vi "QBridge 0MQ weather.vi"() -> (0 "error":errorcluster)   [LabVIEW 2018]
uses:
  <vilib>/addons/zeromq/zmq_socket.lvclass
  <vilib>/addons/zeromq/zmq_context.lvclass
  <vilib>/addons/zeromq/socket_type.ctl
  <vilib>/addons/zeromq/socket_options.ctl
  Global_Telescopio.vi
  <vilib>/addons/zeromq/zeromq.lvlib
panel:
  in  "stop":bool
  # "QBRIDGE ZeroMQ \nSUB Weather"
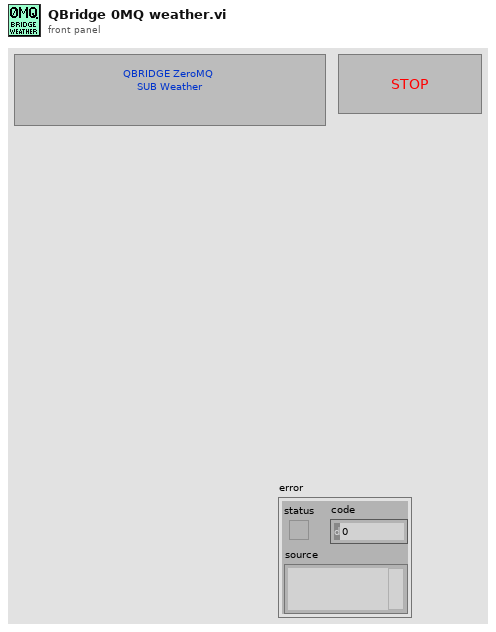
[diagram p1: front panel]
types:
  T1 = typedef "zeromq.lvlib/socket_options.ctl" = enum8{"NONE", "ZMQ_HWM", "<2>", "ZMQ_SWAP", "ZMQ_AFFINITY", "ZMQ_ROUTING_ID", "ZMQ_SUBSCRIBE", "ZMQ_UNSUBSCRIBE", "ZMQ_RATE", "ZMQ_RECOVERY_IVL", "ZMQ_MCAST_LOOP", "ZMQ_SNDBUF", "ZMQ_RCVBUF", "ZMQ_RCVMORE", "ZMQ_FD", "ZMQ_EVENTS", "ZMQ_TYPE", "ZMQ_LINGER", "ZMQ_RECONNECT_IVL", "ZMQ_BACKLOG", "ZMQ_RECOVERY_IVL_MSEC", "ZMQ_RECONNECT_IVL_MAX", "ZMQ_MAXMSGSIZE", "ZMQ_SNDHWM", "ZMQ_RCVHWM", "ZMQ_MULTICAST_HOPS", "<26>", "ZMQ_RCVTIMEO", "ZMQ_SNDTIMEO", "<29>", "<30>", "ZMQ_IPV4ONLY", "ZMQ_LAST_ENDPOINT", "ZMQ_ROUTER_MANDATORY", "ZMQ_TCP_KEEPALIVE", "ZMQ_TCP_KEEPALIVE_CNT", "ZMQ_TCP_KEEPALIVE_IDLE", "ZMQ_TCP_KEEPALIVE_INTVL", "ZMQ_TCP_ACCEPT_FILTER", "ZMQ_IMMEDIATE", "ZMQ_XPUB_VERBOSE", "ZMQ_ROUTER_RAW", "ZMQ_IPV6", "ZMQ_MECHANISM", "ZMQ_PLAIN_SERVER", "ZMQ_PLAIN_USERNAME", "ZMQ_PLAIN_PASSWORD", "ZMQ_CURVE_SERVER", "ZMQ_CURVE_PUBLICKEY", "ZMQ_CURVE_SECRETKEY", "ZMQ_CURVE_SERVERKEY", "ZMQ_PROBE_ROUTER", "ZMQ_REQ_CORRELATE", "ZMQ_REQ_RELAXED", "ZMQ_CONFLATE", "ZMQ_ZAP_DOMAIN", "ZMQ_ROUTER_HANDOVER", "ZMQ_TOS", "ZMQ_IPC_FILTER_PID", "ZMQ_IPC_FILTER_UID", "ZMQ_IPC_FILTER_GID", "ZMQ_CONNECT_ROUTING_ID", "ZMQ_GSSAPI_SERVER", "ZMQ_GSSAPI_PRINCIPAL", "ZMQ_GSSAPI_SERVICE_PRINCIPAL", "ZMQ_GSSAPI_PLAINTEXT", "ZMQ_HANDSHAKE_IVL", "<67>", "ZMQ_SOCKS_PROXY", "ZMQ_XPUB_NODROP", "ZMQ_BLOCKY", "ZMQ_XPUB_MANUAL", "ZMQ_XPUB_WELCOME_MSG", "ZMQ_STREAM_NOTIFY", "ZMQ_INVERT_MATCHING", "ZMQ_HEARTBEAT_IVL", "ZMQ_HEARTBEAT_TTL", "ZMQ_HEARTBEAT_TIMEOUT", "ZMQ_XPUB_VERBOSER", "ZMQ_CONNECT_TIMEOUT", "ZMQ_TCP_MAXRT", "ZMQ_THREAD_SAFE", "<82>", "<83>", "ZMQ_MULTICAST_MAXTPDU", "ZMQ_VMCI_BUFFER_SIZE", "ZMQ_VMCI_BUFFER_MIN_SIZE", "ZMQ_VMCI_BUFFER_MAX_SIZE", "ZMQ_VMCI_CONNECT_TIMEOUT", "ZMQ_USE_FD", "ZMQ_GSSAPI_PRINCIPAL_NAMETYPE", "ZMQ_GSSAPI_SERVICE_PRINCIPAL_NAMETYPE", "ZMQ_BINDTODEVICE", "ZMQ_ZAP_ENFORCE_DOMAIN", "ZMQ_LOOPBACK_FASTPATH", "ZMQ_METADATA", "ZMQ_MULTICAST_LOOP", "ZMQ_ROUTER_NOTIFY"}
  T2 = typedef "zeromq.lvlib/socket_type.ctl" = enum8{"ZMQ_PAIR", "ZMQ_PUB", "ZMQ_SUB", "ZMQ_REQ", "ZMQ_REP", "ZMQ_DEALER", "ZMQ_ROUTER", "ZMQ_PULL", "ZMQ_PUSH", "ZMQ_XPUB", "ZMQ_XSUB", "ZMQ_STREAM", "ZMQ_SERVER", "ZMQ_CLIENT", "ZMQ_RADIO", "ZMQ_DISH", "ZMQ_GATHER", "ZMQ_SCATTER", "ZMQ_DGRAM"}
  T3 = cluster{"broker":string, "version":string, "date":string, "hour":string, "outTemp":string, "hiTemp":string, "lowTemp":string, "outHumidity":string, "dewOut":string, "windSpeed":string, "windDirection":string, "windRun":string, "hiSpeed":string, "hiDir":string, "windChill":string, "heatIndex":string, "THWIndex":string, "THSIndex":string, "pressure":string, "rain":string, "rainRate":string, "solarRad":string, "solarEnergy":string, "hiSolarRad":string, "UVIndex":string, "UVDose":string, "hiUV":string, "headDD":string, "coolDD":string, "inTemp":string, "inHumidity":string, "inHeat":string, "inEMC":string, "inAirDensity":string, "2ndTemp":string, "2ndHumidity":string, "ET":string, "leaf":string, "windSamp":string, "windTx":string, "ISSRecept":string, "dewIn":string, "arcInt":string}
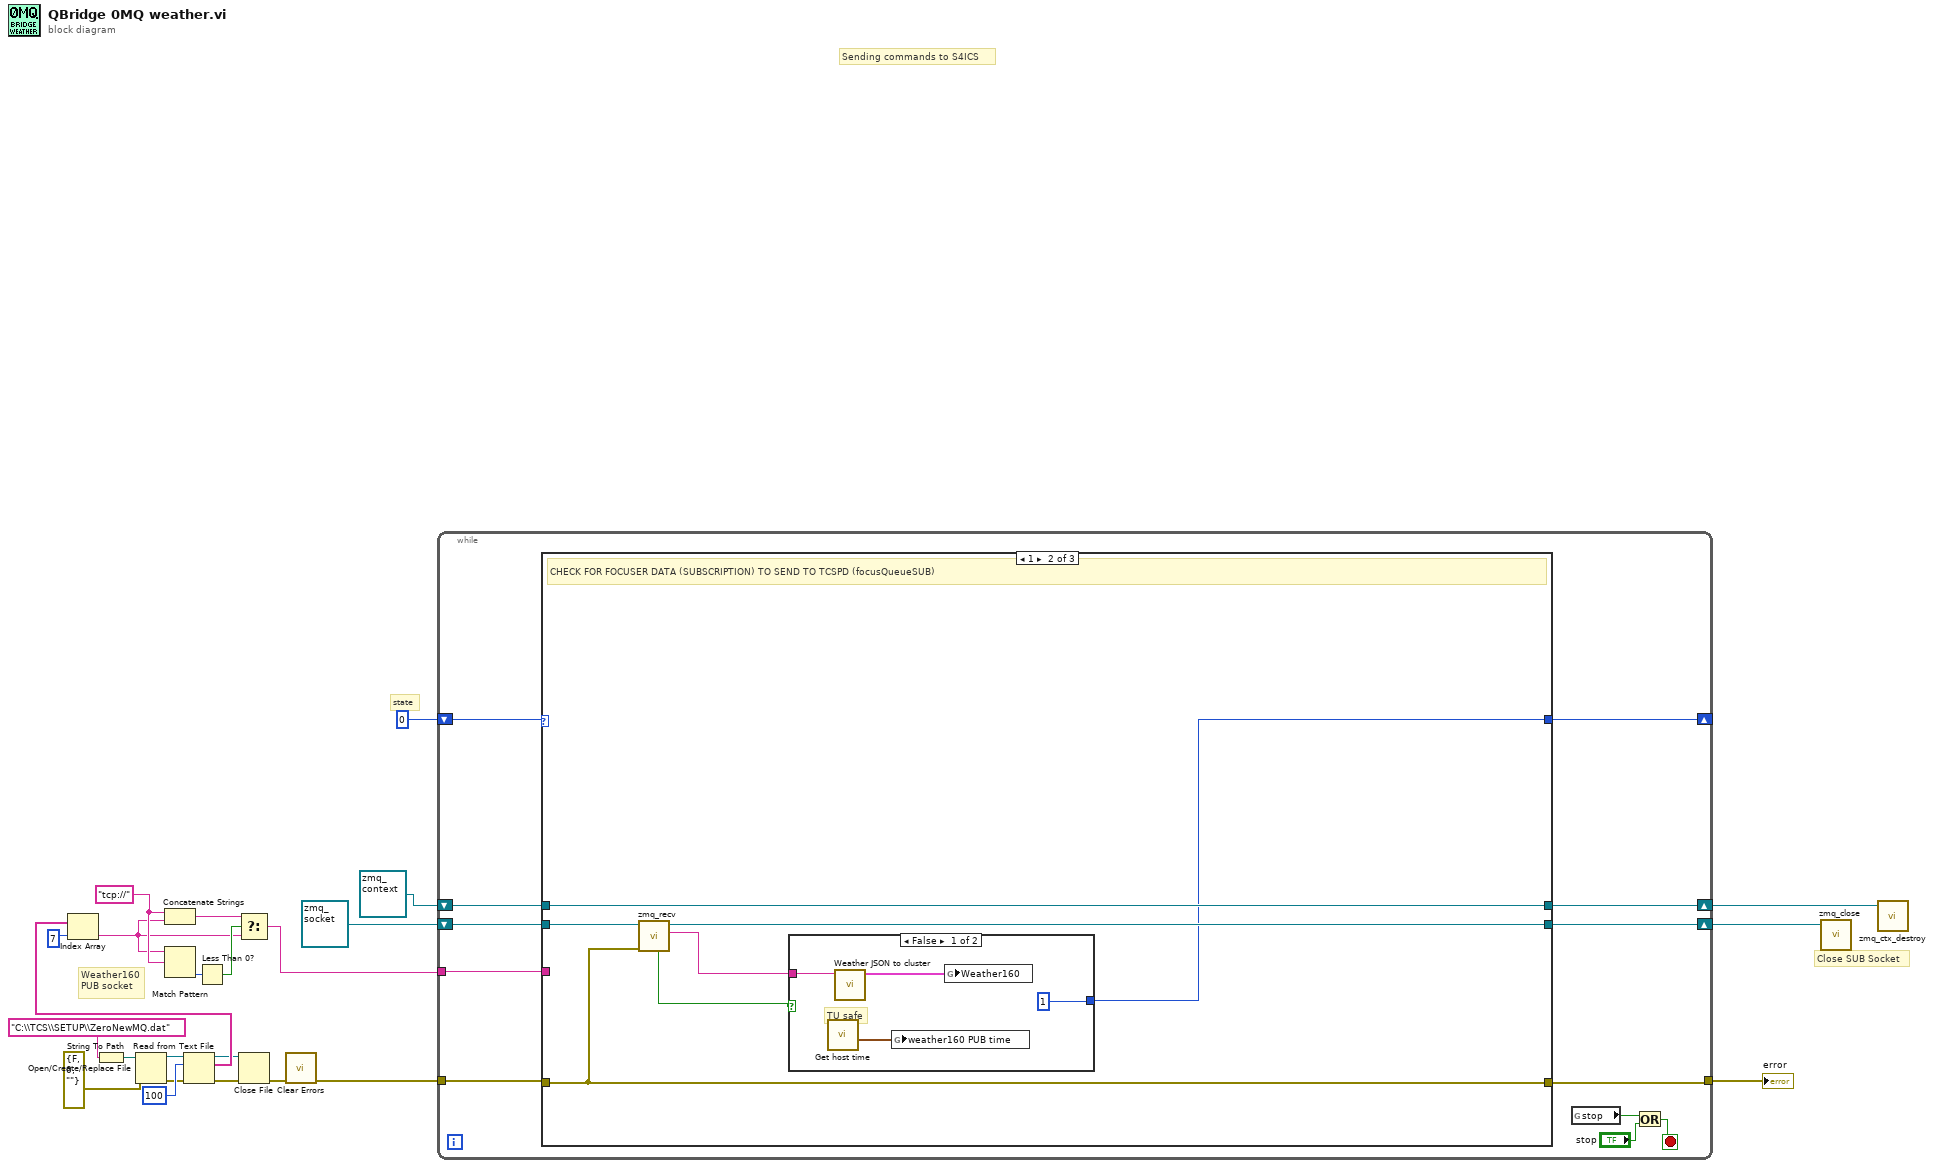
[diagram p0: block diagram]
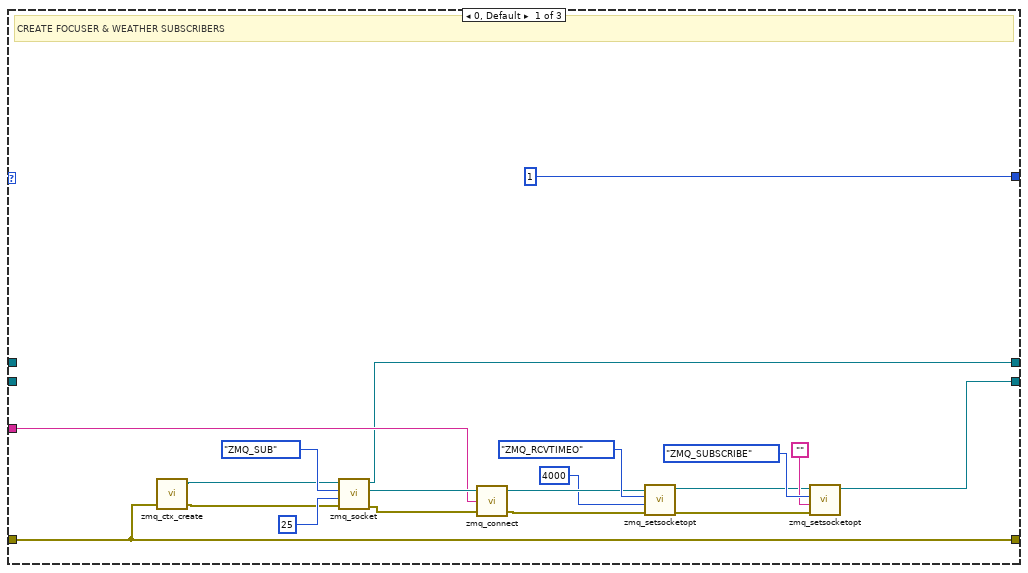
[diagram p2: hidden frame]
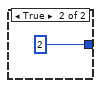
[diagram p3: hidden frame]
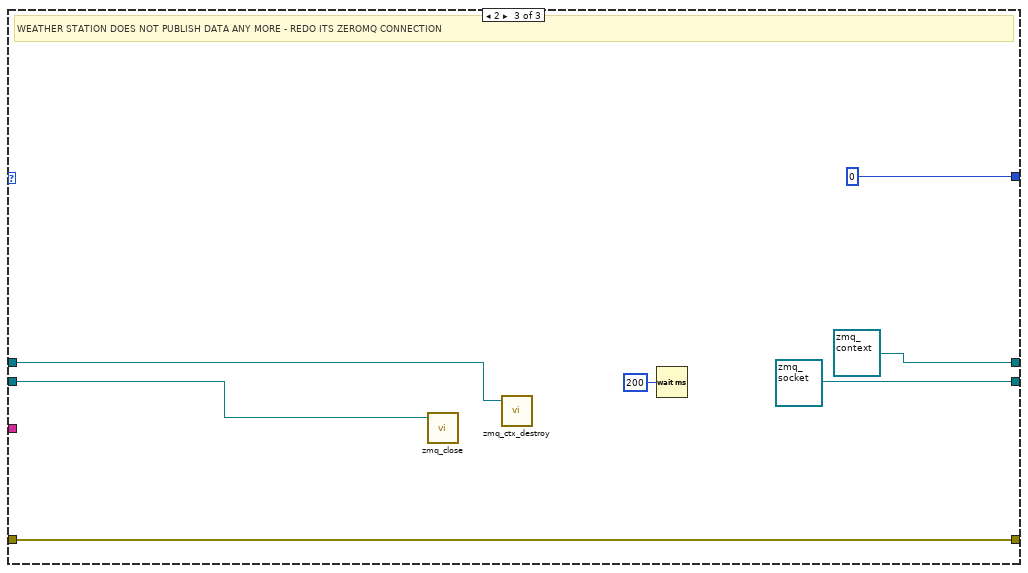
[diagram p4: hidden frame]
diagram:
  w6 = "tcp://"
  # "Close SUB Socket"
  # "Weather160\nPUB socket"
  # "state"
  # "Sending commands to S4ICS"
  n1 = String To Path(string="C:\\TCS\\SETUP\\ZeroNewMQ.dat") -> (path=w22:path)
  n2 = Open/Create/Replace File(file path (use dialog)=w22, error in=errorcluster {"status"=FALSE, "code"=0, "source"=""}) -> (refnum out=w20:refnum<file>, error out=w13:errorcluster)  [unwired: 4 in, 1 out]
  n3 = Read from Text File(file (use dialog)=w20, count=100, error in=w13) -> (refnum out=w16:refnum<file>, text=w18:string[], error out=w11:errorcluster)  [unwired: 1 in, 1 out]
  n4 = Index Array(array=w18, index=7) -> (element=w1:string)
  n5 = Concatenate Strings(w6, w1) -> (w8:string)
  n6 = Match Pattern(string=w1, regular expression=w6) -> (offset past match=w9:i32)  [unwired: 1 in, 3 out]
  n7 = Less Than 0?(x=w9) -> (x < 0?=w7:bool)
  n8 = Select(t=w8, s=w7, f=w1) -> (s? t:f=w5:string)
  n9 = Close File(refnum=w16, error in=w11) -> (error out=w12:errorcluster)  [unwired: 1 out]
  n10 = call <vilib>:"Clear Errors.vi"("error in (no error)"=w12) -> ("error out"=w4:errorcluster)  [unwired: 5 in, 1 out]
  n11 = while {
    shift-right: [w34] -> _
    shift-left: u16 0 -> [w36]
    tunnel: w4 -> [w35]
    tunnel: [w33] -> w23
    shift-right: [w29] -> w10
    shift-left: refnum<class "zmq_socket.lvclass"> refnum ("socket out") -> [w30]
    tunnel: w5 -> [w28]
    shift-right: [w26] -> w2
    shift-left: refnum<class "zmq_context.lvclass"> refnum ("context out") -> [w27]
    stop <- w31 stop-if-true
    n12 = case shown="1" w36 {
      tunnel: w35 -> [w47 w60 w74]
      tunnel: [u16 1 w56 u16 0] -> w34
      tunnel: [w47 w60 w74] -> w33
      tunnel: w30 -> [_ w62 w72]
      tunnel: [w55 w61 refnum<class "zmq_socket.lvclass"> refnum ("socket out")] -> w29
      tunnel: w28 -> [w48 _ _]
      tunnel: w27 -> [_ w58 w71]
      tunnel: [w43 w58 refnum<class "zmq_context.lvclass"> refnum ("context out")] -> w26
      frame 0, Default {
        # "CREATE FOCUSER & WEATHER SUBSCRIBERS"
        n13 = call <vilib>:"zmq_ctx_create.vi"("error in"=w47) -> ("error out"=w44:errorcluster, "context out"=w45:refnum<class "zmq_context.lvclass">)  [unwired: 3 in]
        n14 = call <vilib>:"zmq_socket.vi"("error in"=w44, "linger (ms)"=25, "socket type"=socket_type."ZMQ_SUB", "context in"=w45) -> ("error out"=w53:errorcluster, "socket out"=w54:refnum<class "zmq_socket.lvclass">, "context out"=w43:refnum<class "zmq_context.lvclass">)  [unwired: 1 in]
        n15 = call <vilib>:"zmq_connect.vi"("error in"=w53, "endpoint"=w48, "socket in"=w54) -> ("error out"=w38:errorcluster, "socket out"=w41:refnum<class "zmq_socket.lvclass">)  [unwired: 1 in]
        n16 = call <vilib>:"zmq_setsocketopt.vi"("error in"=w38, "value"=u16 4000, "option"=socket_options."ZMQ_RCVTIMEO", "socket in"=w41) -> ("error out"=w39:errorcluster, "socket out"=w40:refnum<class "zmq_socket.lvclass">)  [unwired: 2 in]
        n17 = call <vilib>:"zmq_setsocketopt.vi"("error in"=w39, "value"="", "option"=socket_options."ZMQ_SUBSCRIBE", "socket in"=w40) -> ("socket out"=w55:refnum<class "zmq_socket.lvclass">)  [unwired: 2 in, 1 out]
      }
      frame 1 {
        # "CHECK FOR FOCUSER DATA (SUBSCRIPTION) TO SEND TO TCSPD (focusQueueSUB)"
        n18 = call <vilib>:"zmq_recv.vi"("error in"=w60, "socket in"=w62) -> ("data"=w59:string, "socket out"=w61:refnum<class "zmq_socket.lvclass">, "timeout?"=w57:bool)  [unwired: 3 in, 2 out]
        n19 = case shown="False" w57 {
          tunnel: w59 -> [w66 _]
          tunnel: [u16 1 u16 2] -> w56
          frame False {
            # "TU safe"
            n20 = call "Get host time.vi"() -> ("BR current time"=w63:timestamp)  [unwired: 8 in, 3 out]
            n21 = call "Weather JSON to cluster.vi"("JSON status"=w66) -> ("Weather160"=w65:T3)  [unwired: 10 in]
            n22 = global write "Global_Telescopio.vi" "weather160 PUB time"(w63) -> ()
            n23 = global write "Global_Telescopio.vi" "Weather160"(w65) -> ()
          }
          frame True {
          }
        }
      }
      frame 2 {
        # "WEATHER STATION DOES NOT PUBLISH DATA ANY MORE - REDO ITS ZEROMQ CONNECTION"
        n24 = call <vilib>:"zmq_close.vi"("socket"=w72) -> ()  [unwired: 4 in, 1 out]
        n25 = call <vilib>:"zmq_ctx_destroy.vi"("context in"=w71) -> ()  [unwired: 4 in, 1 out]
        n26 = Wait (ms)(milliseconds to wait=u32 200) -> ()  [unwired: 1 out]
      }
    }
    n27 = global read "Global_Telescopio.vi" "stop"() -> (w25:bool)
    n28 = Or(x=w25, y="stop") -> (x .or. y?=w31:bool)
  }
  "error" <- w23
  n29 = call <vilib>:"zmq_close.vi"("socket"=w10) -> ()  [unwired: 4 in, 1 out]
  n30 = call <vilib>:"zmq_ctx_destroy.vi"("context in"=w2) -> ()  [unwired: 4 in, 1 out]
